vi "Array Teil.vi"(9 "Spalten":i32, 10 "Zeilen":i32, 11 "Array (Eingang)":string[][](array[string])) -> (2 "Teil Array (Ausgang)":string[][](array[string]), 3 "Array (Ausgang)":string[][](array[string]))   [LabVIEW 2020, in "Linearisierung v2.lvlib" / "SpanEinstellungen.lvlib"]
uses:
  SpanEinstellungen.lvlib
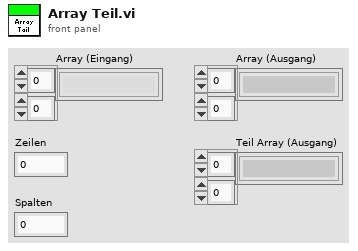
[diagram p1: front panel]
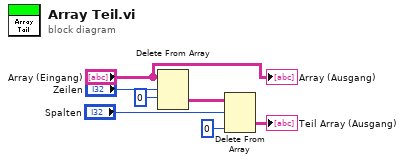
[diagram p0: block diagram]
diagram:
  n1 = Delete From Array(array="Array (Eingang)", length="Zeilen", index (row)=0 ("Index (Zeile)")) -> (deleted portion=w5:string[][])  [unwired: 1 in, 1 out]
  n2 = Delete From Array(array=w5, length="Spalten", index (col)=0 ("Index (Zeile)")) -> (deleted portion=→"Teil Array (Ausgang)":string[][])  [unwired: 1 in, 1 out]
  "Array (Ausgang)" <- "Array (Eingang)"
